vi "Start.vi"(8 "error in":errorcluster) -> (0 "error out":errorcluster)   [LabVIEW 2015, in "PLC.lvlib"]
uses:
  PLC.lvlib
  support/Message Queue/Message Queue.lvlib
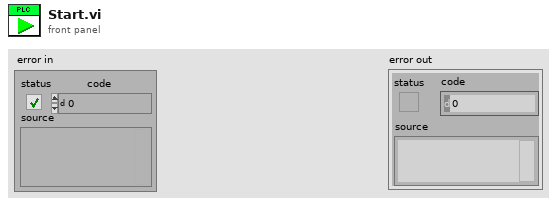
[diagram p1: front panel]
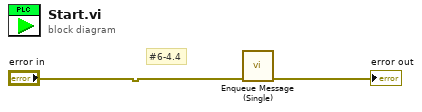
[diagram p0: block diagram]
diagram:
  # "#6-4.4"
  n1 = call "Enqueue Message (Single).vi"("error in (no error)"="error in") -> ("error out"=→"error out":errorcluster)  [unwired: 9 in, 1 out]
